vi "DriveStatus.vi"(0 "Axis In":T2, 11 "error in (no error)":errorcluster) -> (4 "Axis Out":T2, 6 "Status":T1, 15 "error out":errorcluster)   [LabVIEW 2009]
doc: "Get drive status flags."
uses:
  typedefs/AxisSelect_Enum.ctl
  typedefs/Ultra3000/DriveStatus_Cluster.ctl
  typedefs/Ultra3000/Func.ctl
  typedefs/Ultra3000/Cmds.ctl
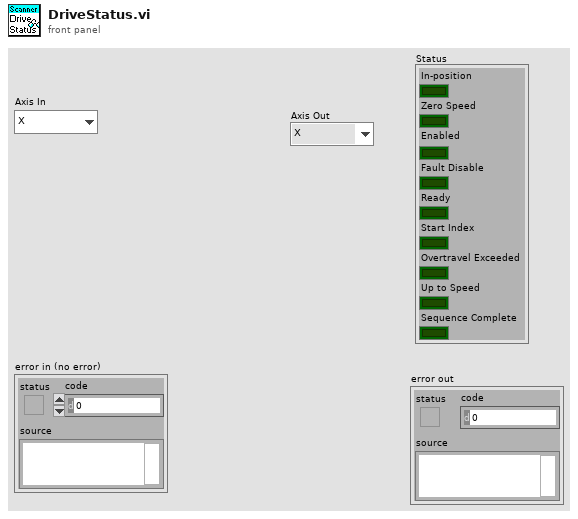
[diagram p1: front panel]
types:
  T1 = typedef "DriveStatus_Cluster.ctl" = cluster{"In-position":bool, "Zero Speed":bool, "Enabled":bool, "Fault Disable":bool, "Ready":bool, "Start Index":bool, "Overtravel Exceeded":bool, "Up to Speed":bool, "Sequence Complete":bool}
  T2 = typedef "AxisSelect_Enum.ctl" = enum16{"X", "Y", "Z", "Axis Space"}
  T3 = typedef "Cmds.ctl" = u16
  T4 = typedef "Func.ctl" = u16
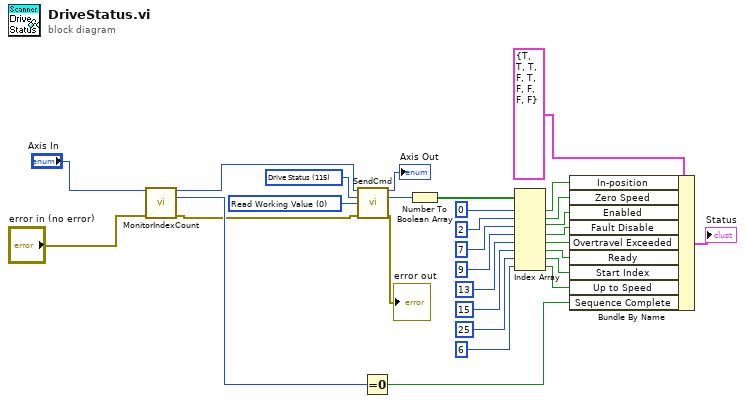
[diagram p0: block diagram]
diagram:
  w28 = T3 115 items=["Drive Status"=115, "Position Command"=128, "Run Status"=117, "Fault Status"=116, "Position Error"=129, "Auto-Start Homing"=196, "Start Homing"=205, "Homing Type"=197, "Motor Position"=126, "Velocity Motor"=133, "Power-Up Status"=1, "Drive Name"=6, "Position Window Size"=22, "Position Window Time"=23, "Zero Speed Limit"=34, "Speed Window Size"=35, "Up to Speed Limit"=37, "Forward Current Limit"=47, "Reverse Current Limit"=48, "Override Mode"=67, "Operation Mode"=90, "Host Control Mode"=97, "Reset Drive"=106, "Drive Enable"=107, "Setpoint Current"=108, "Setpoint Velocity"=109, "Setpoint Acceleration"=110, "Reset Faults"=111, "Position Comparator"=349, "Postition Comparator Polarity"=350, "Position Rollover Enable"=404, "Baud Rate"=80, "Frame Format"=81, "Drive Address"=82, "Broadcast Address"=83, "Auto-start Indexing"=88, "Start Index"=112, "Host Index"=184, "Index Type"=174, "Index Dist/Pos"=175, "Index Reg Dist"=176, "Index Velocity"=177, "Index Acceleration"=178, "Index Deceleration"=179, "Index Dwell"=180, "Index Count"=181, "Index Termination"=182, "Index Pointer"=183, "Index Abort Deceleration"=185, "Positive Soft Pos Limit"=216, "Define Home"=113, "Negative Soft Pos Limit"=217] ("Command")
  w29 = T4 0 items=["Read Working Value", "Write Working Value", "Read Non-Volatile Value", "Write Non-Volatile and Woring Value", "Copy Non-Volatile Value to Working Value", "Copy Working Value to Non-Volatile Value", "Read Default Value", "Copy Default Value to Non-Volatile and Working Values", "Read Min Value", "Read Max Value", "Read Array Index Min", "Read Array Index Max"] ("Function")
  n1 = call "MonitorIndexCount.vi"("Axis In"="Axis In", "error in (no error)"="error in (no error)") -> ("Axis Out"=w5:T2, "Index Count"=w7:u16, "error out"=w6:errorcluster)  [unwired: 11 in]
  n2 = call "SendCmd.vi"("Axis In"=w5, "Command"=w28, "Function"=w29, "error in (no error)"=w6) -> ("Axis Out"=→"Axis Out":T2, "Data"=w27:i32, "error out"=→"error out":errorcluster)  [unwired: 8 in, 1 out]
  n3 = Equal To 0?(x=w7) -> (x = 0?=w3:bool)
  n4 = Number To Boolean Array(number=w27) -> (Boolean array=w26:bool[])
  n5 = Index Array(array=w26, index #1=0 ("index"), index #2=2 ("index"), index #3=7 ("index"), index #4=9 ("index"), index #5=13 ("index"), index #6=15 ("index"), index #7=25 ("index"), index #8=6 ("index")) -> (element #1=w24:bool, element #2=w22:bool, element #3=w20:bool, element #4=w18:bool, element #5=w17:bool, element #6=w13:bool, element #7=w12:bool, element #8=w10:bool)
  n6 = Bundle By Name(cluster=T1 {"In-position"=TRUE, "Zero Speed"=TRUE, "Enabled"=TRUE, "Fault Disable"=FALSE, "Ready"=TRUE, "Start Index"=FALSE, "Overtravel Exceeded"=FALSE, "Up to Speed"=FALSE, "Sequence Complete"=FALSE} ("Status"), "In-position"=w24, "Zero Speed"=w22, "Enabled"=w20, "Fault Disable"=w18, "Overtravel Exceeded"=w17, "Ready"=w13, "Start Index"=w12, "Up to Speed"=w10, "Sequence Complete"=w3) -> (→"Status":T1)
